vi "hydrolysis_reactor.vi"(2 "#":i16, 4 "Dataflow In":errorcluster) -> (1 "Dataflow Out":errorcluster)   [LabVIEW 2019]
uses:
  lib/libSimulationControl/libSimulationControl.lvlib
panel:
  out "prior_active_element":string
  # "*******************************************************************\nBiogas Plant Control\n\nAuthor: Paul Zügel\nGCSC-Frankfurt am Main 2020\n\n*******************************************************************"
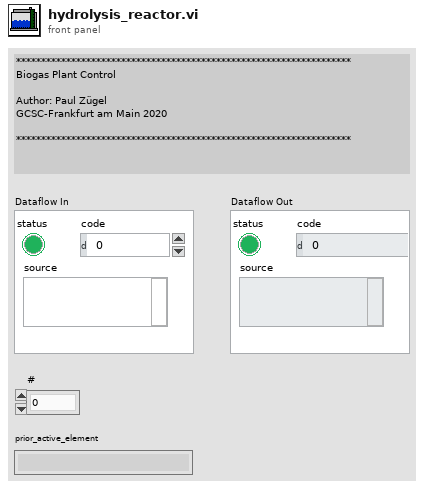
[diagram p1: front panel]
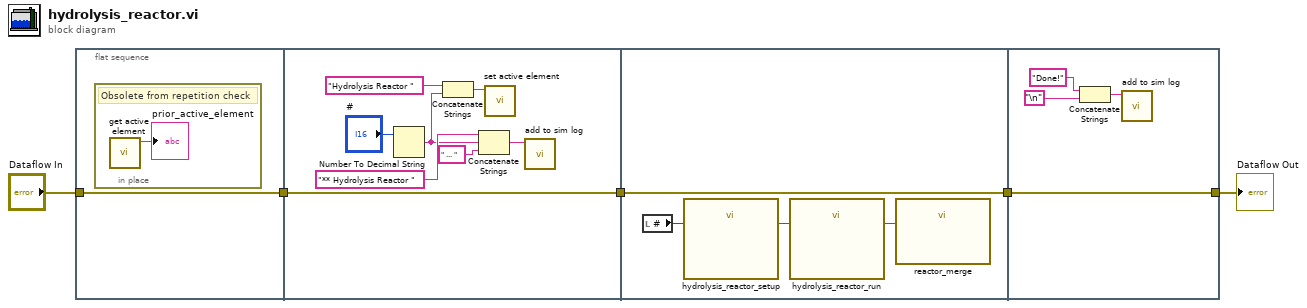
[diagram p0: block diagram]
diagram:
  n1 = flat-sequence {
    tunnel: "Dataflow In" -> [w6]
    tunnel: [w6] -> w2
    tunnel: [w15] -> w4
    tunnel: w2 -> [w15]
    tunnel: [w19] -> w1
    tunnel: w4 -> [w19]
    tunnel: [w23] -> w3
    tunnel: w1 -> [w23]
    frame #0 {
      n2 = in-place {
        # "Obsolete from repetition check"
        n3 = call "get active element.vi"() -> ("active_element"=→"prior_active_element":string)  [unwired: 10 in, 1 out]
      }
    }
    frame #1 {
      n4 = Number To Decimal String(number="#") -> (decimal integer string=w11:string)  [unwired: 1 in]
      n5 = Concatenate Strings("Hydrolysis Reactor " ("elem"), w11) -> (w13:string)
      n6 = Concatenate Strings("** Hydrolysis Reactor " ("string"), w11, " ... " ("string")) -> (w9:string)
      n7 = call "set active element.vi"("elem"=w13) -> ()  [unwired: 10 in, 1 out]
      n8 = call "add to sim log.vi"("log"=w9) -> ()  [unwired: 10 in, 1 out]
    }
    frame #2 {
      n9 = local read "#"() -> (w18:i16)
      n10 = call "hydrolysis_reactor_setup.vi"("#"=w18) -> ("spec_file"=w17:path)  [unwired: 10 in]
      n11 = call "hydrolysis_reactor_run.vi"("spec_file"=w17) -> ("hydrolysis_path"=w16:path)  [unwired: 10 in]
      n12 = call "reactor_merge.vi"("reactor_path"=w16) -> ()  [unwired: 11 in]
    }
    frame #3 {
      n13 = Concatenate Strings("Done!" ("string"), "\n") -> (w20:string)
      n14 = call "add to sim log.vi"("log"=w20) -> ()  [unwired: 10 in, 1 out]
    }
  }
  "Dataflow Out" <- w3
